vi "Autosize All MultiListbox Columns (Uniform Text).vi"(6 "IngoreCols(Empty as default)":i32[](array[numeric]), 8 "error in (no error)":errorcluster, 10 "Array":string[][](array[string]), 11 "Control in":refnum<vi>) -> (0 "error out":errorcluster)   [LabVIEW 2014, in "csm-tool-support.lvlib"]
doc: "This VI resizes each column of the table specified by Table Ref based on the widest entry of the column. Additionally, if Resize Table? is TRUE, the VI will set the table width based on the number of populated columns."
uses:
  csm-tool-support.lvlib
  7259d3e2-cfed-496a-970d-f2c931f09757.vi
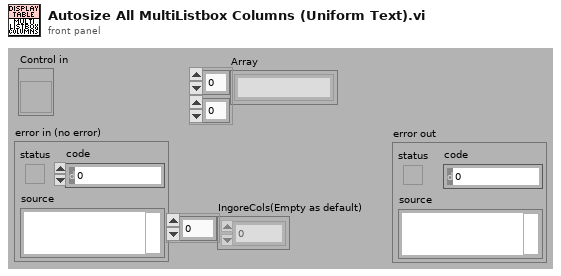
[diagram p1: front panel]
types:
  T1 = enum16{"User-specified Font", "Application Font", "System Font", "Dialog Font"}
  T2 = cluster{"Font Name:":string, "Size":i16, "Strikeout?":bool, "Italic?":bool, "Underline?":bool, "Outline?":bool, "Shadow?":bool, "Bold?":bool}
  T3 = cluster{"left":i16, "top":i16, "right":i16, "bottom":i16}
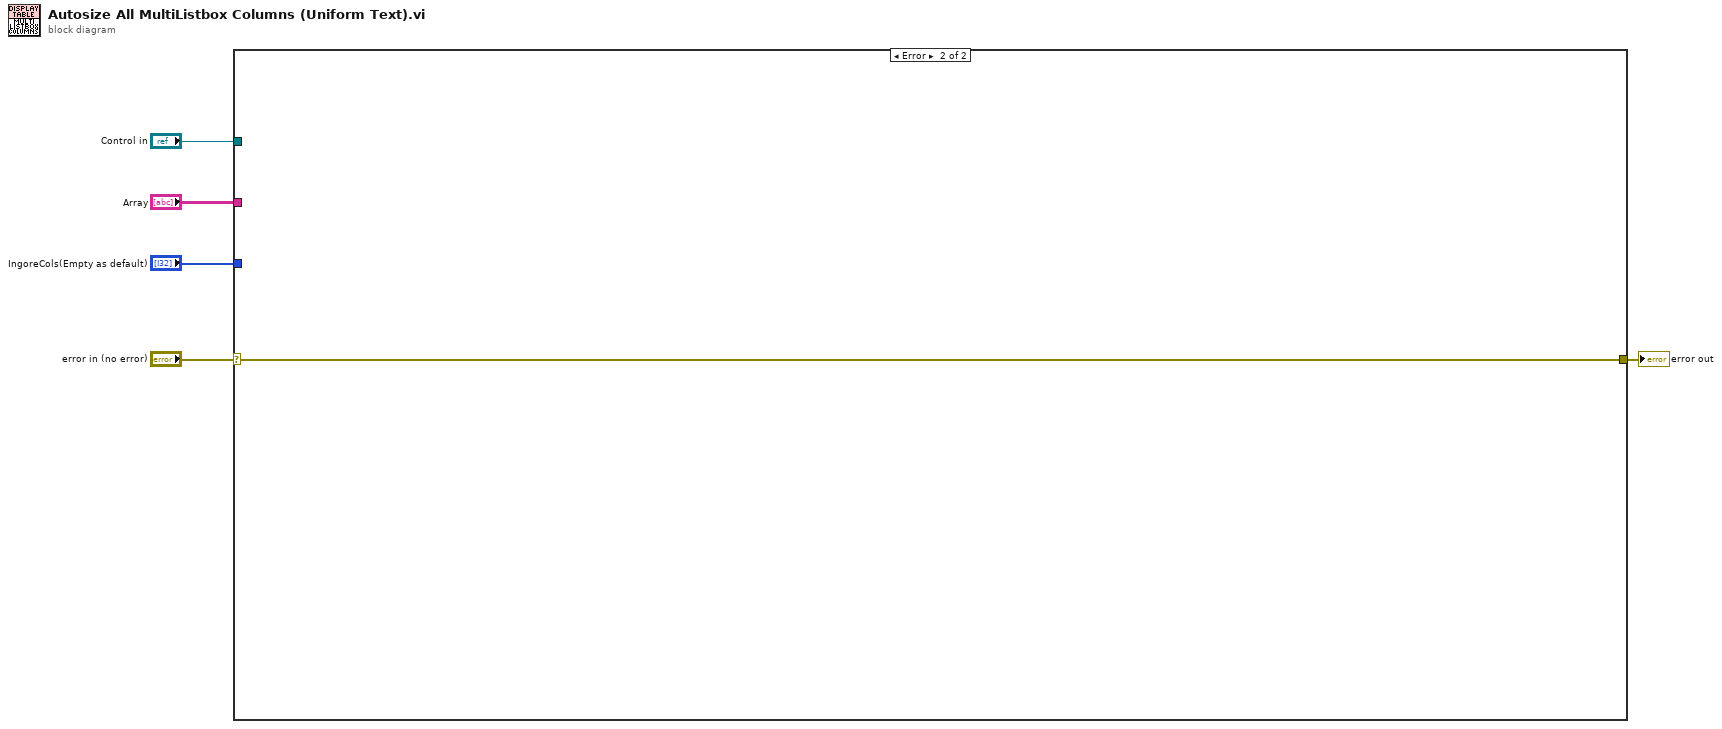
[diagram p0: block diagram]
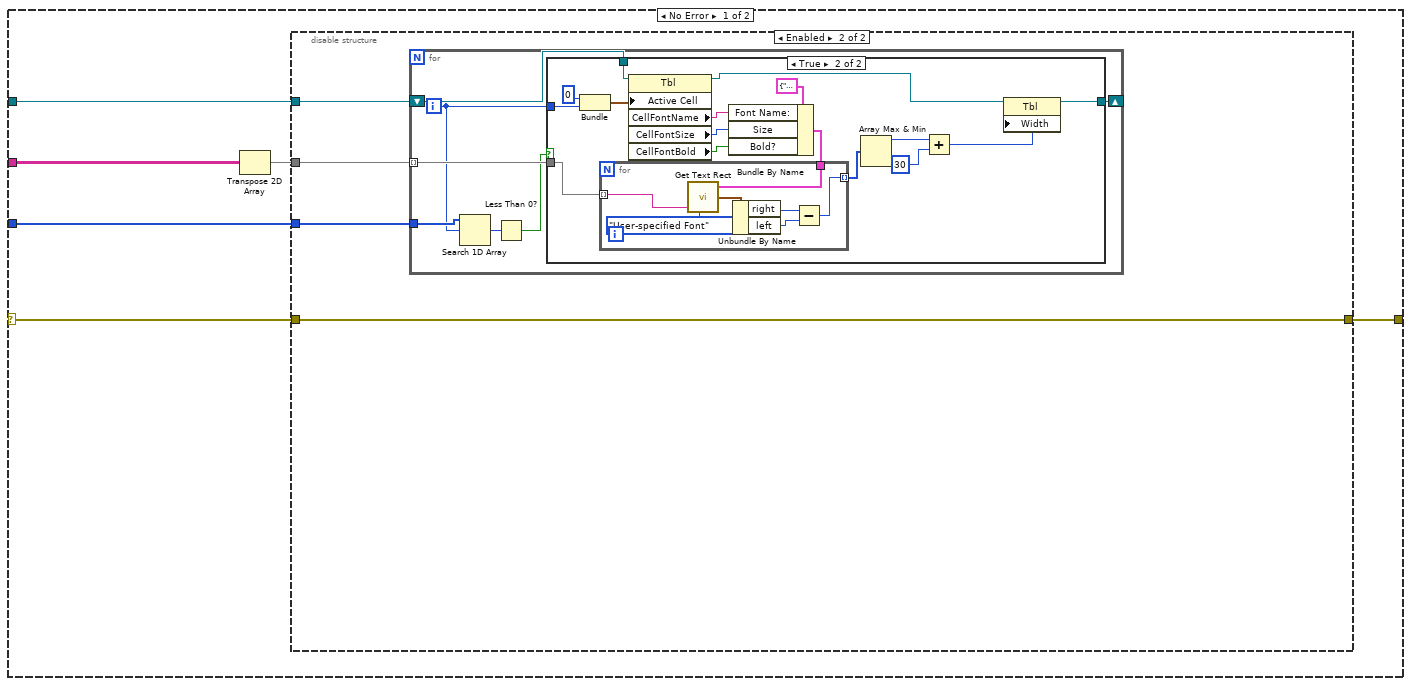
[diagram p2: hidden frame]
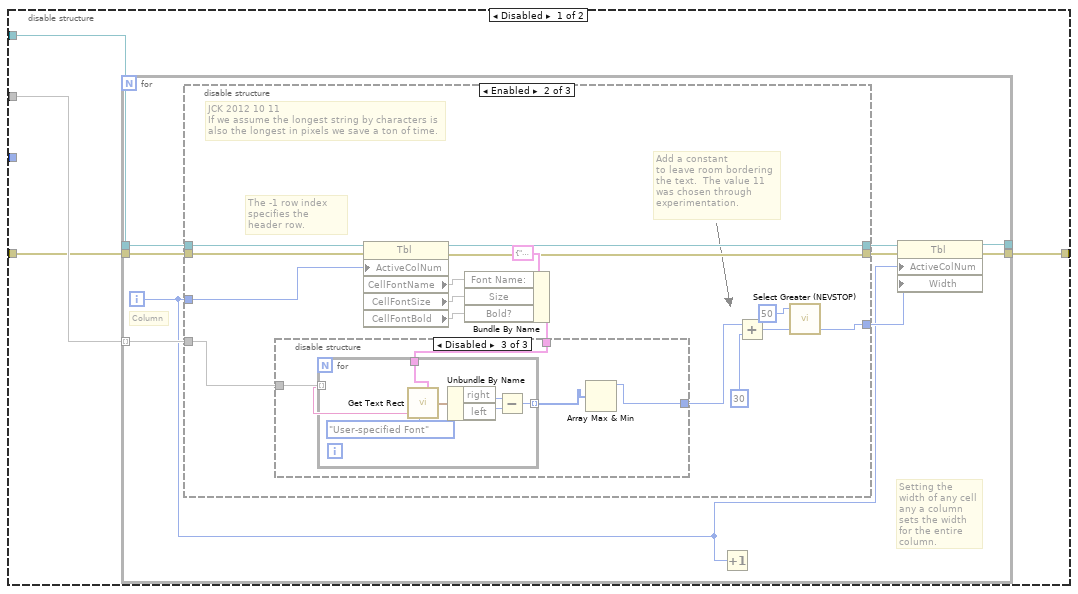
[diagram p3: hidden frame]
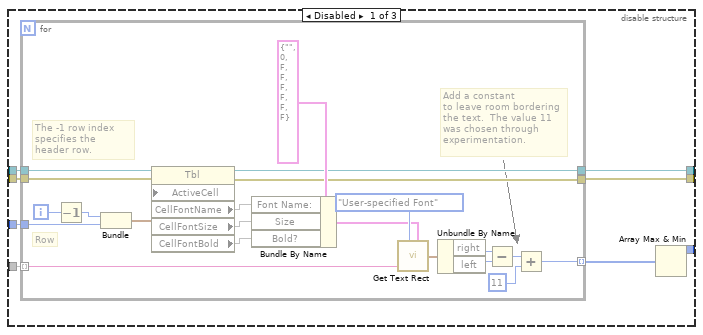
[diagram p4: hidden frame]
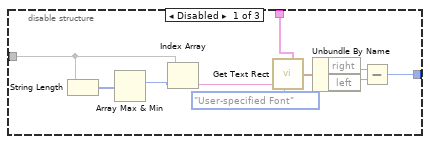
[diagram p5: hidden frame]
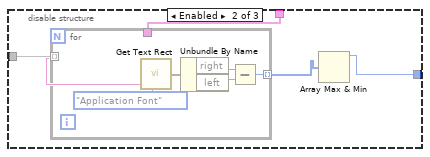
[diagram p6: hidden frame]
diagram:
  n1 = case shown="Error" "error in (no error)" {
    selector: "error in (no error)" -> [w10 w137]
    tunnel: "Control in" -> [w9 _]
    tunnel: [w8 w137] -> w3
    tunnel: "Array" -> [w7 _]
    tunnel: "IngoreCols(Empty as default)" -> [w6 _]
    frame No Error {
      n2 = Transpose 2D Array(2D array=w7) -> (transposed array=w11:string[][])
      n3 = disable-structure shown="Enabled" {
        disable-tunnel: w9 -> [w16 w105]
        disable-tunnel: w11 -> [w15 w104]
        disable-tunnel: w10 -> [w14 w103]
        disable-tunnel: [w12 w103] -> w8
        disable-tunnel: w6 -> [_ w102]
        frame Disabled {
          n4 = for {
            tunnel: w15 -> [w25] mode=indexing
            tunnel: w16 -> [w24]
            tunnel: w14 -> [w23]
            tunnel: [w19] -> w12
            tunnel: [w18] -> w13
            i -> [w17]
            # "Setting the width of any cell any a column sets the width for the entire column."
            # "Column"
            n5 = disable-structure shown="Enabled" {
              disable-tunnel: w25 -> [w33 w63 _]
              disable-tunnel: w24 -> [w32 w62 _]
              disable-tunnel: w23 -> [w30 w61 _]
              disable-tunnel: [w29 w60 _] -> w22
              disable-tunnel: [w28 w59 _] -> w21
              disable-tunnel: [w27 w56 _] -> w20
              disable-tunnel: w17 -> [w26 w57 _]
              frame Disabled {
                n6 = for {
                  tunnel: w33 -> [w46] mode=indexing
                  tunnel: w32 -> [w54]
                  tunnel: w26 -> [w53]
                  tunnel: [w35] -> w31 mode=indexing
                  tunnel: w30 -> [w40]
                  tunnel: [w39] -> w28
                  tunnel: [w38] -> w29
                  i -> [w42]
                  # "The -1 row index specifies the header row."
                  # "Add a constant\nto leave room bordering the text.  The value 11 was chosen through experimentation."
                  # "Row"
                  n7 = Decrement(x=w42) -> (x-1=w41:i32)
                  n8 = Bundle(w41, w53) -> (w52:cluster{i32, i32})  [unwired: 1 in]
                  n9 = property class="Tbl"(reference=w54, error in=w40, "ActiveCell"=w52) -> (reference out=w38:refnum<vi>, error out=w39:errorcluster, "CellFontName"=w50, "CellFontSize"=w36, "CellFontBold"=w49)
                  n10 = Bundle By Name(cluster=T2 {"Font Name:"="", "Size"=0, "Strikeout?"=FALSE, "Italic?"=FALSE, "Underline?"=FALSE, "Outline?"=FALSE, "Shadow?"=FALSE, "Bold?"=FALSE} ("[user-specified font]"), "Font Name:"=w50, "Size"=w36, "Bold?"=w49) -> (w47:T2)
                  n11 = call <vilib>:"Get Text Rect.vi"("desired font(Application)"=T1."User-specified Font", "text"=w46, "[user-specified font]"=w47) -> ("rect"=w45:T3)  [unwired: 6 in]
                  n12 = Unbundle By Name(w45) -> ("right"=w44:i16, "left"=w43:i16)
                  n13 = Subtract(x=w44, y=w43) -> (x-y=w37:i16)
                  n14 = Add(x=w37, y=i16 11) -> (x+y=w35:i16)
                }
                n15 = Array Max & Min(array=w31) -> (max value=w27:i16)  [unwired: 3 out]
              }
              frame Enabled {
                # "JCK 2012 10 11\nIf we assume the longest string by characters is also the longest in pixels we save a ton of time."
                # "The -1 row index specifies the header row."
                # "Add a constant\nto leave room bordering the text.  The value 11 was chosen through experimentation."
                n16 = property class="Tbl"(reference=w62, error in=w61, "ActiveColNum"=w57) -> (reference out=w60:refnum<vi>, error out=w59:errorcluster, "CellFontName"=w65, "CellFontSize"=w69, "CellFontBold"=w66)
                n17 = Bundle By Name(cluster=T2 {"Font Name:"="", "Size"=0, "Strikeout?"=FALSE, "Italic?"=FALSE, "Underline?"=FALSE, "Outline?"=FALSE, "Shadow?"=FALSE, "Bold?"=FALSE} ("[user-specified font]"), "Font Name:"=w65, "Size"=w69, "Bold?"=w66) -> (w67:T2)
                n18 = disable-structure shown="Disabled" {
                  disable-tunnel: [w79 w81 w91] -> w68
                  disable-tunnel: w67 -> [w75 w84 w94]
                  disable-tunnel: w63 -> [w73 w83 w93]
                  frame Disabled {
                    n19 = String Length(string=w73) -> (length=w80:i32[])
                    n20 = Array Max & Min(array=w80) -> (max index (indices)=w72:i32)  [unwired: 3 out]
                    n21 = Index Array(array=w73, index=w72) -> (element=w71:string)
                    n22 = call <vilib>:"Get Text Rect.vi"("desired font(Application)"=T1."User-specified Font", "text"=w71, "[user-specified font]"=w75) -> ("rect"=w76:T3)  [unwired: 6 in]
                    n23 = Unbundle By Name(w76) -> ("right"=w77:i16, "left"=w78:i16)
                    n24 = Subtract(x=w77, y=w78) -> (x-y=w79:i16)
                  }
                  frame Enabled {
                    n25 = for {
                      tunnel: [w90] -> w82 mode=indexing
                      tunnel: w84 -> [_]
                      tunnel: w83 -> [w85] mode=indexing
                      n26 = call <vilib>:"Get Text Rect.vi"("desired font(Application)"=T1."Application Font", "text"=w85) -> ("rect"=w87:T3)  [unwired: 7 in]
                      n27 = Unbundle By Name(w87) -> ("right"=w88:i16, "left"=w89:i16)
                      n28 = Subtract(x=w88, y=w89) -> (x-y=w90:i16)
                    }
                    n29 = Array Max & Min(array=w82) -> (max value=w81:i16)  [unwired: 3 out]
                  }
                  frame Disabled {
                    n30 = for {
                      tunnel: [w101] -> w92 mode=indexing
                      tunnel: w94 -> [w97]
                      tunnel: w93 -> [w95] mode=indexing
                      n31 = call <vilib>:"Get Text Rect.vi"("desired font(Application)"=T1."User-specified Font", "text"=w95, "[user-specified font]"=w97) -> ("rect"=w98:T3)  [unwired: 6 in]
                      n32 = Unbundle By Name(w98) -> ("right"=w99:i16, "left"=w100:i16)
                      n33 = Subtract(x=w99, y=w100) -> (x-y=w101:i16)
                    }
                    n34 = Array Max & Min(array=w92) -> (max value=w91:i16)  [unwired: 3 out]
                  }
                }
                n35 = Add(x=w68, y=i16 30) -> (x+y=w58:i16)
                n36 = call "Select Greater (NEVSTOP)"("A"=i16 50 ("y"), "B"=w58) -> ("lesser"=w56:i16)  [unwired: 3 in]
              }
              frame Disabled {
              }
            }
            n37 = Increment(x=w17) -> ()  [unwired: 1 out]
            n38 = property class="Tbl"(reference=w22, error in=w21, "ActiveColNum"=w17, "Width"=w20) -> (reference out=w18:refnum<vi>, error out=w19:errorcluster)
          }
        }
        frame Enabled {
          n39 = for {
            tunnel: w104 -> [w112] mode=indexing
            shift-right: [w110] -> _
            shift-left: w105 -> [w111]
            tunnel: w102 -> [w109]
            i -> [w108]
            n40 = Search 1D Array(1D array=w109, element=w108) -> (index of element=w107:i32)  [unwired: 1 in]
            n41 = Less Than 0?(x=w107) -> (x < 0?=w106:bool)
            n42 = case shown="True" w106 {
              tunnel: w112 -> [_ w129]
              tunnel: w108 -> [_ w119]
              tunnel: w111 -> [w113 w120]
              tunnel: [w113 w116] -> w110
              frame False {
              }
              frame True {
                n43 = Bundle(0, w119) -> (w115:cluster{i32, i32})  [unwired: 1 in]
                n44 = property class="Tbl"(reference=w120, "Active Cell"=w115) -> (reference out=w117:refnum<vi>, "CellFontName"=w124:string, "CellFontSize"=w122:u32, "CellFontBold"=w123:bool)  [unwired: 1 in, 1 out]
                n45 = Bundle By Name(cluster=T2 {"Font Name:"="", "Size"=0, "Strikeout?"=FALSE, "Italic?"=FALSE, "Underline?"=FALSE, "Outline?"=FALSE, "Shadow?"=FALSE, "Bold?"=FALSE} ("[user-specified font]"), "Font Name:"=w124, "Size"=w122, "Bold?"=w123) -> (w118:T2)
                n46 = for {
                  tunnel: w129 -> [w136] mode=indexing
                  tunnel: [w132] -> w128 mode=indexing
                  tunnel: w118 -> [w131]
                  n47 = call <vilib>:"Get Text Rect.vi"("desired font(Application)"=T1."User-specified Font", "text"=w136, "[user-specified font]"=w131) -> ("rect"=w135:T3)  [unwired: 6 in]
                  n48 = Unbundle By Name(w135) -> ("right"=w134:i16, "left"=w133:i16)
                  n49 = Subtract(x=w134, y=w133) -> (x-y=w132:i16)
                }
                n50 = Array Max & Min(array=w128) -> (max value=w125:i16)  [unwired: 3 out]
                n51 = Add(x=w125, y=i16 30) -> (x+y=w126:i16)
                n52 = property on="Property Node" class="Tbl"(reference=w117, "Width"=w126) -> (reference out=w116:refnum<vi>)  [unwired: 1 in, 1 out]
              }
            }
          }
        }
      }
    }
    frame Error {
    }
  }
  "error out" <- w3
